vi "(SubVI) Set Scanrate and Pull_YCC.vi"(0 "toward+ ?\nT=+, F=-":bool, 1 "Start From  (um)":dbl min=0.0 max=100.0 step=0.5 format="%.3f", 2 "axis":u32=1, 3 "scan rate  (um/s)":dbl=2.0 format="%.3f", 4 "waiting time per point (ms)\nrange from 5ms to 0.167 ms":dbl=5.0, 5 "range  (um)":dbl=2.0 min=0.0 max=100.0 step=0.5 format="%.3f") -> (6 "True rate?":bool, 7 "traveling time (s)":dbl, 8 "step size (nm)":dbl)   [LabVIEW 2014]
uses:
  (Global) Current handle and LaserPower_YCC.vi
  MCL-dll-Labview 32-bit/Madlib.dll
panel:
  out "s? t:f":dbl
  out "x/y":dbl
  out "true scan rate (um/s)":dbl
  out "size(s)":i32
  out "Waveform Graph":dbl[](graph)
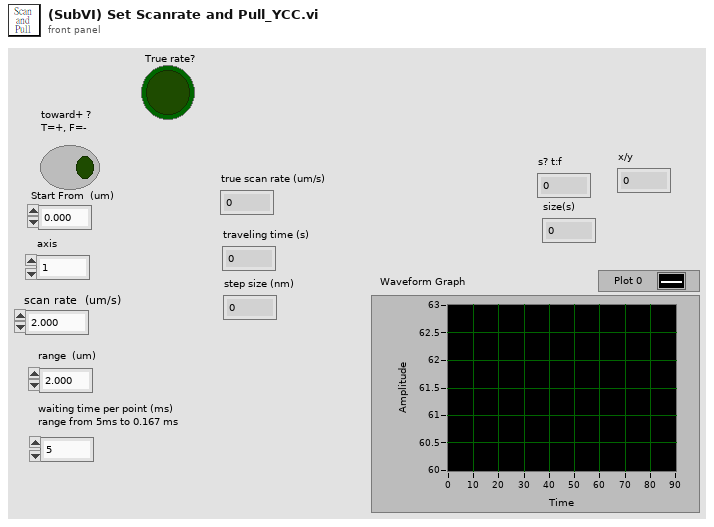
[diagram p1: front panel]
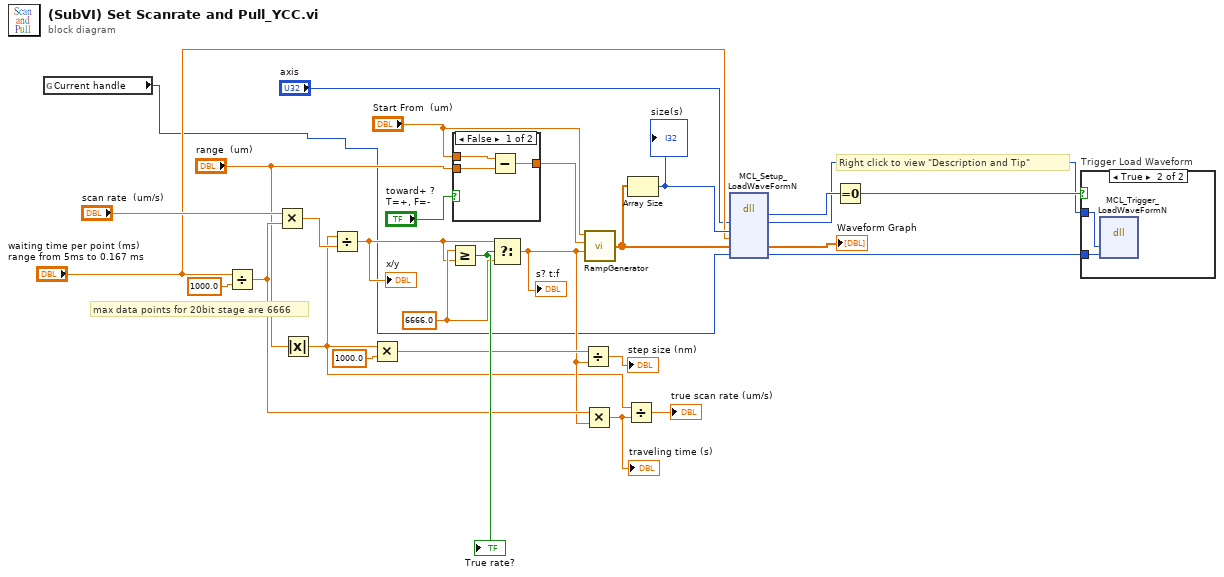
[diagram p0: block diagram]
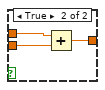
[diagram p2: hidden frame]
diagram:
  w9 = 6666.0 ("t")
  # "max data points for 20bit stage are 6666"
  # "Right click to view \"Description and Tip\""
  n1 = global read "(Global) Current handle and LaserPower_YCC.vi" "Current handle"() -> (w1:i32)
  n2 = Divide(x="waiting time per point (ms)\nrange from 5ms to 0.167 ms", y=1000.0) -> (x/y=w14:dbl)
  n3 = Multiply(x="scan rate  (um/s)", y=w14) -> (x*y=w27:dbl)
  n4 = Absolute Value(x="range  (um)") -> (abs(x)=w7:dbl)
  n5 = Divide(x=w7, y=w27) -> (x/y=w8:dbl)
  "x/y" <- w8
  n6 = Multiply(x=w7, y=1000.0) -> (x*y=w12:dbl)
  n7 = Greater Or Equal?(x=w9, y=w8) -> (x >= y?=w17:bool)
  "True rate?" <- w17
  n8 = case shown="False" "toward+ ?\nT=+, F=-" {
    tunnel: "Start From  (um)" -> [w31 w34]
    tunnel: "range  (um)" -> [w30 w33]
    tunnel: [w29 w32] -> w5
    frame False {
      n9 = Subtract(x=w31, y=w30) -> (x-y=w29:dbl)
    }
    frame True {
      n10 = Add(x=w34, y=w33) -> (x+y=w32:dbl)
    }
  }
  n11 = Select(t=w8, s=w17, f=w9) -> (s? t:f=w11:dbl)
  "s? t:f" <- w11
  n12 = Divide(x=w12, y=w11) -> (x/y=→"step size (nm)":dbl)
  n13 = Multiply(x=w14, y=w11) -> (x*y=w13:dbl)
  "traveling time (s)" <- w13
  n14 = call "RampGenerator.vi"("Number of Positions"=w11, "End  (um)"=w5, "Start  (um)"="Start From  (um)") -> ("Array"=w22:dbl[])  [unwired: 1 in]
  n15 = Divide(x=w7, y=w13) -> (x/y=→"true scan rate (um/s)":dbl)
  n16 = Array Size(array=w22) -> (size(s)=w23:i32)
  "size(s)" <- w23
  n17 = dll-call lib="C:/Users/OT-hwlab/Desktop/YCC's OT/Main-Stage-Based/SubVI-Stage-Based/MCL-dll-Labview 32-bit/MADLib.dll" fn="MCL_Setup_LoadWaveFormN" label="Setup WF Load"("axis"="axis", "DataPoints"=w23, "milliseconds"="waiting time per point (ms)\nrange from 5ms to 0.167 ms", "waveform"=w22, "handle"=w1) -> (w21:i32, "axis"=w20:u32, "waveform"=→"Waveform Graph":dbl[], "handle"=w19:i32)  [unwired: 5 in, 2 out]
  n18 = Equal To 0?(x=w21) -> (x = 0?=w24:bool)
  n19 = case "Trigger Load Waveform" shown="True" w24 {
    tunnel: w20 -> [_ w36]
    tunnel: w19 -> [_ w35]
    frame False {
    }
    frame True {
      n20 = dll-call lib="C:/Users/OT-hwlab/Desktop/YCC's OT/Main-Stage-Based/SubVI-Stage-Based/MCL-dll-Labview 32-bit/MADLib.dll" fn="MCL_Trigger_LoadWaveFormN" ("Trigger Load Waveform")("axis"=w36, "handle"=w35) -> ()  [unwired: 6 in, 2 out]
    }
  }
